vi "PH_Sequencer.PC SetGateGenGUIElements.vi"(0 "i ref in":refnum<vi>, 5 "error in (no error)":errorcluster) -> (14 "i ref out":refnum<vi>, 19 "error out":errorcluster)   [LabVIEW 2009]
doc: "This VI sets the GateGen GUI elements depending on the sequencer state machine state."
uses:
  PH_Sequencer.lvlib
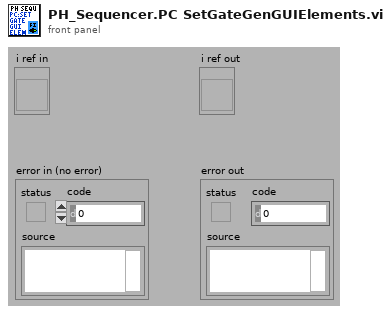
[diagram p1: front panel]
types:
  T1 = typedef "PH_Sequencer.lvlib/PH_Sequencer.i attribute.ctl" = cluster{"GUI Refs":cluster{"Main Off":refnum<vi>, "Fire":refnum<vi>, "Status":refnum<vi>, "Ready":refnum<vi>, "Waiting Time":refnum<vi>, "Timeout":refnum<vi>, "SMs ok":refnum<vi>, "PP DP Ready":refnum<vi>, "Sequencer SM State":refnum<vi>, "PP PA Ready":refnum<vi>, "Calorimeter":refnum<vi>, "Beamline Ready":refnum<vi>, "Clear Beamline":refnum<vi>, "Linkage PPMA Rods":refnum<vi>, "Linkage Current PA":refnum<vi>, "Linkage Current MA":refnum<vi>, "Linkage PPMA Rods 2":refnum<vi>, "Linkage PPMA Rods 3":refnum<vi>, "Linkage Current MA 2":refnum<vi>, "Linkage Current MA 3":refnum<vi>, "PP Booster Ready":refnum<vi>, "PP FR Ready":refnum<vi>, "Timing Ready":refnum<vi>, "State Timing":refnum<vi>, "Force Timing":refnum<vi>, "PSDB Shot Comment":refnum<vi>, "State PA Backreflection":refnum<vi>, "Beamline Z6 Ready":refnum<vi>, "Clear Z6 Beamline":refnum<vi>, "Sequence length":refnum<vi>, "Timing Mode":refnum<vi>, "Slow Trigger Settings":refnum<vi>, "Experiment Description":refnum<vi>, "State PSDB":refnum<vi>, "PSDB Ready":refnum<vi>, "Set PSDB Settings":refnum<vi>, "Get PSDB Info":refnum<vi>, "Take Snapshot":refnum<vi>, "Shottype":refnum<vi>, "Experiment":refnum<vi>, "PA Energy":refnum<vi>, "MA Energy":refnum<vi>, "MA Gain":refnum<vi>}, "Status Info":cluster{"Machine Status":T2, "WaitingTime":i32, "Timeout":bool}, "Readyness":cluster{"Ready to shot":bool, "PP DP Ready":bool, "PPPA Ready":bool, "BL Ready":bool, "PP Booster Ready":bool, "PP FR Ready":bool, "Timing Ready":bool, "BL Z6 Ready":bool, "PSDBReady":bool}, "Instancenames":cluster{"PPMA Rods":string, "PP Current Meas":string, "Beamline":string, "PA Backrefl Meas":string, "Beamline Z6":string}, "Data to read":bool, "Calorimeter":cluster{"Instancename":string, "On":bool, "linked":bool}, "Linkage":cluster{"PPMA Rods":bool, "PP Current Meas":bool, "Beamline":bool, "PA Backrefl Meas":bool, "Beamline Z6":bool}, "PU Info":T3[], "HV Info":T4[], "PSU Info":T5[], "Refs PU on":refnum<vi>[], "Refs Set Voltage PU":refnum<vi>[], "Refs State PU":refnum<vi>[], "Refs State SM PU":refnum<vi>[], "Refs Waiting Time PU":refnum<vi>[], "Refs TO SM PU":refnum<vi>[], "Refs Voltage PU":refnum<vi>[], "Timing":cluster{"Instance":string, "linked":bool, "Status":T2, "Timing Mode":T6, "Slow Trigger Settings":T7, "Info available":cluster{"ext SlowTrigger":bool, "T2":bool, "Mode":bool, "Delay Slow Trigger":bool}}, "GUI Manager Path":string, "Service ID R2S":i32, "PSDB":cluster{"Controller Instance":string, "Controller Status":T2, "Controller linked":bool, "Settings acknowledged":bool, "Current Experiment ID":i16, "Current Shot Type":i16, "Current Comment":string, "Remember Settings":bool, "Write 2 early":bool}, "PSDB Data":cluster{"Main Off?":bool, "Sequence Length":dbl, "Sequence startet":timestamp}, "Beamline":refnum<vi>[], "Powermeter":cluster{"PA":cluster{"Instance":string, "Energy [J]":dbl, "in use":bool}, "MA":cluster{"Instance":string, "Energy [J]":dbl, "in use":bool}, "MA Gain":dbl}}
  T2 = typedef "Status.ctl" = i16
  T3 = typedef "PH_Sequencer.lvlib/PH_Sequencer.PU Info.ctl" = cluster{"Instancename":string, "PU on":bool, "State":T2, "Waiting time":i32, "Set Voltage":dbl, "State SM":string, "Timeout SM":string, "linked":bool}
  T4 = typedef "PH_Sequencer.lvlib/PH_Sequencer.HV Meas Info.ctl" = cluster{"Instancename":string, "linked":bool, "Tagname Meas Voltage":string}
  T5 = typedef "PH_Sequencer.lvlib/PH_Sequencer.PSU Info.ctl" = cluster{"Instancename":string, "linked":bool, "Tagname Applied Voltage":string}
  T6 = typedef "PH_Timing.lvlib/PH_Timing.Timing Mode.ctl" = cluster{"T2 [s]":i16, "Modeselector":enum32{"10 Hz", "0.5 Hz", "Shot"}}
  T7 = typedef "PH_Timing.lvlib/PH_Timing.Slow Trigger Settings.ctl" = cluster{"Delay [ms]":dbl, "externally triggered?":bool}
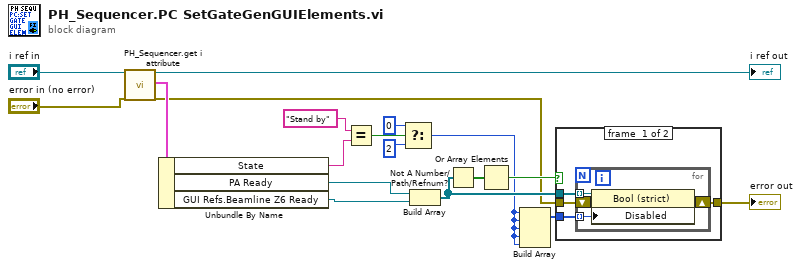
[diagram p0: block diagram]
diagram:
  n1 = call "PH_Sequencer.get i attribute.vi"("i ref in"="i ref in", "error in (no error)"="error in (no error)") -> ("i ref out"=→"i ref out":refnum<vi>, "i attribute"=w14:T1, "error out"=w6:errorcluster)  [unwired: 15 in]
  n2 = Unbundle By Name(w14) -> ("State"=w2:string, "PA Ready"=w4:refnum<vi>, "GUI Refs.Beamline Z6 Ready"=w1:refnum<vi>)
  n3 = Equal?(x="Stand by", y=w2) -> (x = y?=w12:bool)
  n4 = Select(t=0, s=w12, f=2 ("element")) -> (s? t:f=w3:i32)
  n5 = Build Array(w4, w1) -> (w9:refnum<vi>[])
  n6 = Not A Number/Path/Refnum?(number/path/refnum=w9) -> (NaN/Path/Refnum?=w11:bool[])
  n7 = Or Array Elements(Boolean array=w11) -> (logical OR=w10:bool)
  n8 = Build Array(w3, w3, w3, w3, w3) -> (w8:i32[])
  n9 = case shown="False" w10 {
    tunnel: w9 -> [w22 _]
    tunnel: w8 -> [w21 _]
    tunnel: w6 -> [w20 w27]
    tunnel: [w19 w27] -> w15
    frame #0 {
      n10 = for {
        tunnel: w22 -> [w26] mode=indexing
        tunnel: w21 -> [w25] mode=indexing
        shift-right: [w23] -> w19
        shift-left: w20 -> [w24]
        n11 = property class="Bool (strict)"(reference=w26, error in=w24, "Disabled"=w25) -> (error out=w23:errorcluster)  [unwired: 1 out]
      }
    }
    frame #1 {
    }
  }
  "error out" <- w15
